vi "Locate Corner with known height.vi"(6 "Corner Type":string="Mat", 7 "picture":refnum<vi>, 8 "error in":errorcluster, 9 "Hover":dbl=130.0, 10 "Height":dbl=-105.0, 11 "color":string="Mat") -> (0 "error out":errorcluster, 2 "Robot Pose":cluster{"X":dbl, "Y":dbl, "Z":dbl, "A":dbl}, 5 "picture":picture)   [LabVIEW 2013]
uses:
  ROS/Code/SubVIs/BaxterSide.ctl
  <vilib>/Analysis/baseanly.llb/Mean (DBL).vi
  Arm Globals.vi
  Prim/Fwd Kenimatics - array.vi
  <vilib>/Analysis/Matrix/Numeric/Multiply/Multiply - RM,RM.vi
  ROS/Code/Console/Servers/ServerSubs/(nist) Arm Globals.vi
  <vilib>/Analysis/Matrix/NI_Matrix.lvlib
  <vilib>/Analysis/NI_AALBase.lvlib
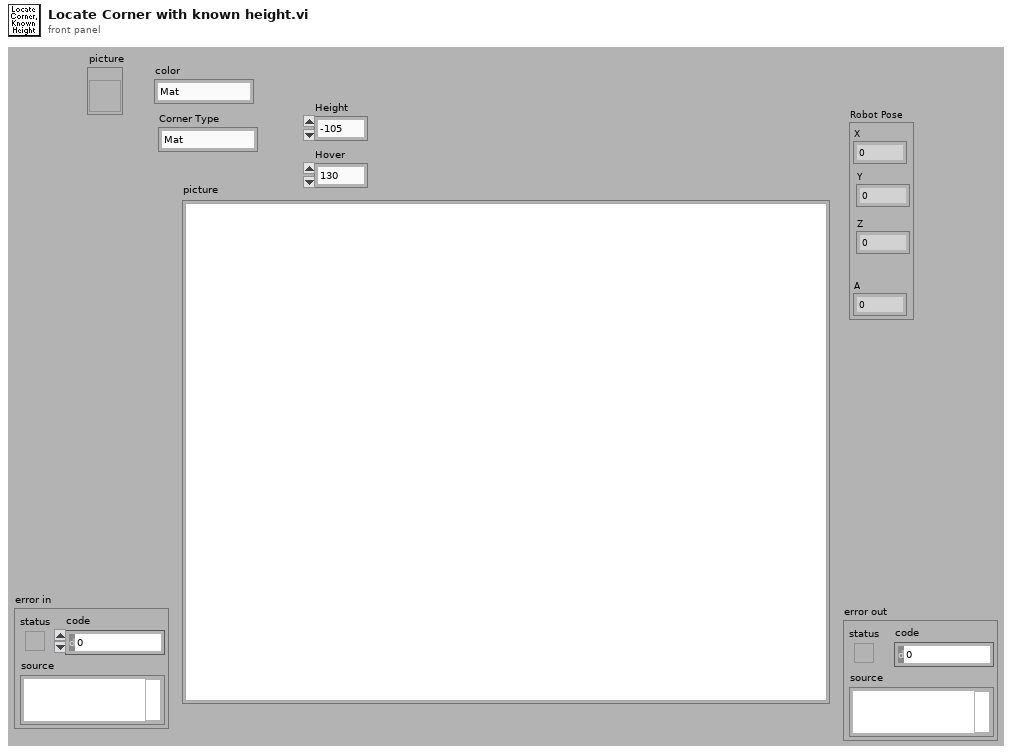
[diagram p1: front panel]
types:
  T1 = typedef "BaxterSide.ctl" = enum16{"left", "right"}
  T2 = enum16{"User-specified Font", "Application Font", "System Font", "Dialog Font"}
  T3 = cluster{"Font Name:":string, "Size":i16, "Strikeout?":bool, "Italic?":bool, "Underline?":bool, "Outline?":bool, "Shadow?":bool, "Bold?":bool}
  T4 = cluster{"X":dbl, "Y":dbl, "Z":dbl, "O":dbl, "A":dbl, "T":dbl}
  T5 = cluster{"left":i16, "top":i16, "right":i16, "bottom":i16}
  T6 = typedef "LVBoundsTypeDef.ctl" = cluster{"Width":u32, "Height":u32}
  T7 = typedef "NI_Matrix.lvlib/RealMatrix.ctl" = dbl[][]
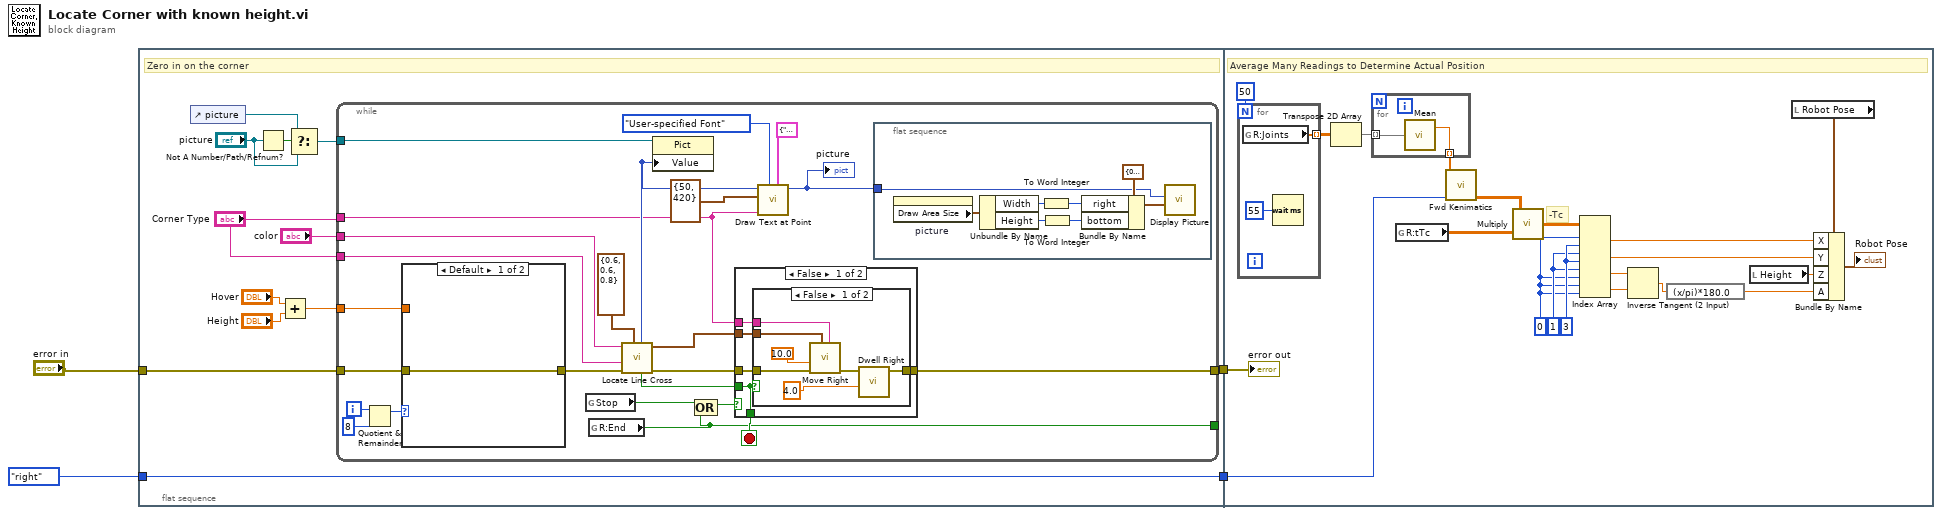
[diagram p0: block diagram]
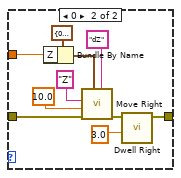
[diagram p2: hidden frame]
diagram:
  n1 = flat-sequence {
    tunnel: [w16] -> w4
    tunnel: [w10] -> w3
    tunnel: BaxterSide."right" ("Side") -> [w10]
    tunnel: "error in" -> [w8]
    tunnel: w4 -> [w81]
    tunnel: w3 -> [w80]
    frame #0 {
      # "Zero in on the corner"
      n2 = control-ref of="picture"() -> (w14:refnum<vi>)
      n3 = Not A Number/Path/Refnum?(number/path/refnum="picture") -> (NaN/Path/Refnum?=w12:bool)
      n4 = Add(x="Hover", y="Height") -> (x+y=w5:dbl)
      n5 = Select(t=w14, s=w12, f="picture") -> (s? t:f=w11:refnum<vi>)
      n6 = while {
        tunnel: w8 -> [w27]
        tunnel: [w39] -> w16
        tunnel: "color" -> [w36]
        tunnel: w11 -> [w32]
        tunnel: [w30] -> _
        tunnel: "Corner Type" -> [w24]
        tunnel: "Corner Type" -> [w29]
        tunnel: w5 -> [w26]
        i -> [w19]
        stop <- w33 stop-if-true
        n7 = Quotient & Remainder(x=w19, y=8) -> (x-y*floor(x/y)=w17:i32)  [unwired: 1 out]
        n8 = case shown="Default" w17 {
          tunnel: [w41 w44] -> w28
          tunnel: w27 -> [w41 w43]
          tunnel: w26 -> [_ w42]
          frame Default {
          }
          frame 0 {
            n9 = Bundle By Name(cluster=T4 {"X"=0.0, "Y"=0.0, "Z"=0.0, "O"=0.0, "A"=0.0, "T"=0.0} ("Goal Axes"), "Z"=w42) -> (w49:T4)
            n10 = call "Move Right.vi"("Label"="dZ" ("Location"), "Goal"=w49, "error in"=w43, "Speed"=10.0, "Mask"="Z") -> ("error out"=w47:errorcluster)  [unwired: 2 in, 4 out]
            n11 = call "Dwell Right.vi"("Wait Time"=3.0 ("wait time"), "error in"=w47) -> ("error out"=w44:errorcluster)  [unwired: 9 in]
          }
        }
        n12 = global read "Arm Globals.vi" "Stop"() -> (w37:bool)
        n13 = global read "Arm Globals.vi" "R:End"() -> (w30:bool)
        n14 = call "Locate Line Cross.vi"("Tolerance"=cluster{"x":dbl, "y":dbl, "a":dbl} {"x"=0.6, "y"=0.6, "a"=0.8}, "error in"=w28, "Type"=w29, "color"=w36) -> ("error out"=w40:errorcluster, "result"=w38:T4, "Close"=w34:bool, "picture"=w25:picture)  [unwired: 2 in, 2 out]
        n15 = property class="Pict"(reference=w32, "Value"=w25) -> ()  [unwired: 1 in, 2 out]
        n16 = Compound Arithmetic op=OR(w37, w30) -> (w35:bool)
        n17 = case shown="False" w35 {
          selector: w35 -> [_ w73]
          tunnel: w34 -> [w61 _]
          tunnel: w40 -> [w64 w74]
          tunnel: [w63 w74] -> w39
          tunnel: w38 -> [w62 _]
          tunnel: [w61 w73] -> w33
          tunnel: w24 -> [w60 _]
          frame False {
            n18 = case shown="False" w61 {
              tunnel: w64 -> [w71 w72]
              tunnel: [w66 w72] -> w63
              tunnel: w62 -> [w67 _]
              tunnel: w60 -> [w68 _]
              frame False {
                n19 = call "Move Right.vi"("Label"=w68, "Goal"=w67, "error in"=w71, "Speed"=10.0) -> ("error out"=w70:errorcluster)  [unwired: 3 in, 4 out]
                n20 = call "Dwell Right.vi"("Wait Time"=4.0, "error in"=w70) -> ("error out"=w66:errorcluster)  [unwired: 9 in]
              }
              frame True {
              }
            }
          }
          frame True {
          }
        }
        n21 = call <vilib>:"Draw Text at Point.vi"("[user-specified font]"=T3 {"Font Name:"="Arial Black", "Size"=60, "Strikeout?"=FALSE, "Italic?"=FALSE, "Underline?"=FALSE, "Outline?"=FALSE, "Shadow?"=FALSE, "Bold?"=TRUE}, "desired font(Application)"=T2."User-specified Font", "text"=w24, "origin"=cluster{"x":i16, "y":i16} {"x"=50, "y"=420}, "picture"=w25) -> ("new picture"=w20:picture)  [unwired: 5 in, 1 out]
        "picture" <- w20
        n22 = flat-sequence {
          tunnel: w20 -> [w53]
          frame #0 {
            n23 = property on="picture" class="Pict"() -> ("Draw Area Size"=w59:T6)  [unwired: 2 in, 2 out]
            n24 = Unbundle By Name(w59) -> ("Width"=w56:u32, "Height"=w57:u32)
            n25 = To Word Integer(number=w56) -> (16bit integer=w55:i16)
            n26 = To Word Integer(number=w57) -> (16bit integer=w54:i16)
            n27 = Bundle By Name(cluster=T5 {"left"=0, "top"=0, "right"=642, "bottom"=534} ("rect"), "right"=w55, "bottom"=w54) -> (w52:T5)
            n28 = call "Display Picture.vi"("rect"=w52, "picture"=w53) -> ()  [unwired: 9 in, 1 out]
          }
        }
      }
    }
    frame #1 {
      w89 = 1 ("index (row)")
      w94 = 3 ("index (col)")
      w88 = 0 ("index (row)")
      # "-Tc"
      # "Average Many Readings to Determine Actual Position"
      n29 = for {
        N: 50 -> [_]
        tunnel: [w99] -> w92 mode=indexing
        n30 = global read "(nist) Arm Globals.vi" "R:Joints"() -> (w99:dbl[])
        n31 = Wait (ms)(milliseconds to wait=u32 55) -> ()  [unwired: 1 out]
      }
      n32 = Transpose 2D Array(2D array=w92) -> (transposed array=w91:dbl[][])
      n33 = for {
        tunnel: w91 -> [w97] mode=indexing
        tunnel: [w96] -> w90 mode=indexing
        n34 = call-poly <vilib>:"Mean.vi"("X"=w97) -> ("mean"=w96:dbl)  [unwired: 1 out]
      }
      n35 = global read "Arm Globals.vi" "R:tTc"() -> (w75:T7)
      n36 = call-poly "Fwd Kenimatics.vi"("Side"=w80, "Joints"=w90) -> ("Matrix"=w77:T7)  [unwired: 8 in, 1 out]
      n37 = call-poly <vilib>:"Multiply.vi"("Real Matrix B"=w75, "Real Matrix A"=w77) -> ("A * B"=w76:T7)
      n38 = Index Array(array=w76, index (row) #1=w88, index (col) #1=w94, index (row) #2=w89, index (col) #2=w94, index (row) #3=w89, index (col) #3=w88, index (row) #4=w88, index (col) #4=w88) -> (element #1=w78:dbl, element #2=w79:dbl, element #3=w87:dbl, element #4=w86:dbl)
      n39 = Inverse Tangent (2 Input)(1:w86, 2:w87) -> (0:w95:dbl)
      n40 = expression code="(x/pi)*180.0" ("radians to degrees")(w95) -> (w82:dbl)
      n41 = local read "Height"() -> (w83:dbl)
      n42 = local read "Robot Pose"() -> (w85:cluster{"X":dbl, "Y":dbl, "Z":dbl, "A":dbl})
      n43 = Bundle By Name(cluster=w85, "X"=w78, "Y"=w79, "Z"=w83, "A"=w82) -> (→"Robot Pose":cluster{"X":dbl, "Y":dbl, "Z":dbl, "A":dbl})
      "error out" <- w81
    }
  }
